vi "Frame Get i.vi"(8 "error in (no error)":errorcluster, 11 "IDE simple in":refnum<class "LF2R IDE.lvclass">) -> (0 "error out":errorcluster, 1 "<i> Data":T1, 2 "Iindex":u32, 3 "IDE simple out":refnum<class "LF2R IDE.lvclass">)   [LabVIEW 2018, in "LF2R IDE.lvlib" / "LF2R IDE.lvclass"]
uses:
  LF2R IDE.lvclass
  Frame Analizer/frame i data.ctl
  LF2R IDE.lvclass/LF2R IDE.ctl
  Frame Analizer/Data Parser.lvclass
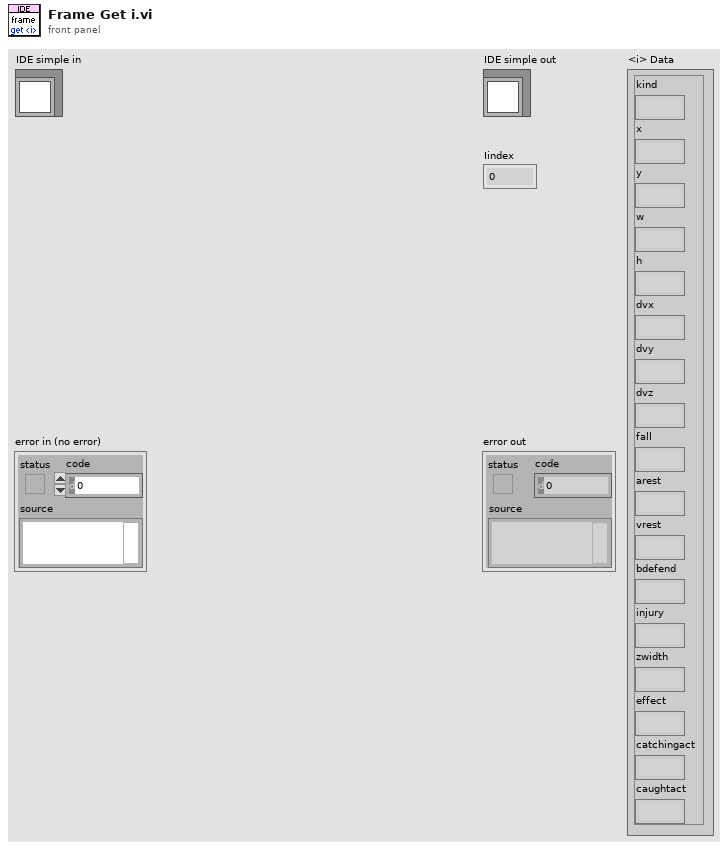
[diagram p1: front panel]
types:
  T1 = typedef "Data Parser.lvclass/frame i data.ctl" = cluster{"kind":string, "x":string, "y":string, "w":string, "h":string, "dvx":string, "dvy":string, "dvz":string, "fall":string, "arest":string, "vrest":string, "bdefend":string, "injury":string, "zwidth":string, "effect":string, "catchingact":string, "caughtact":string}
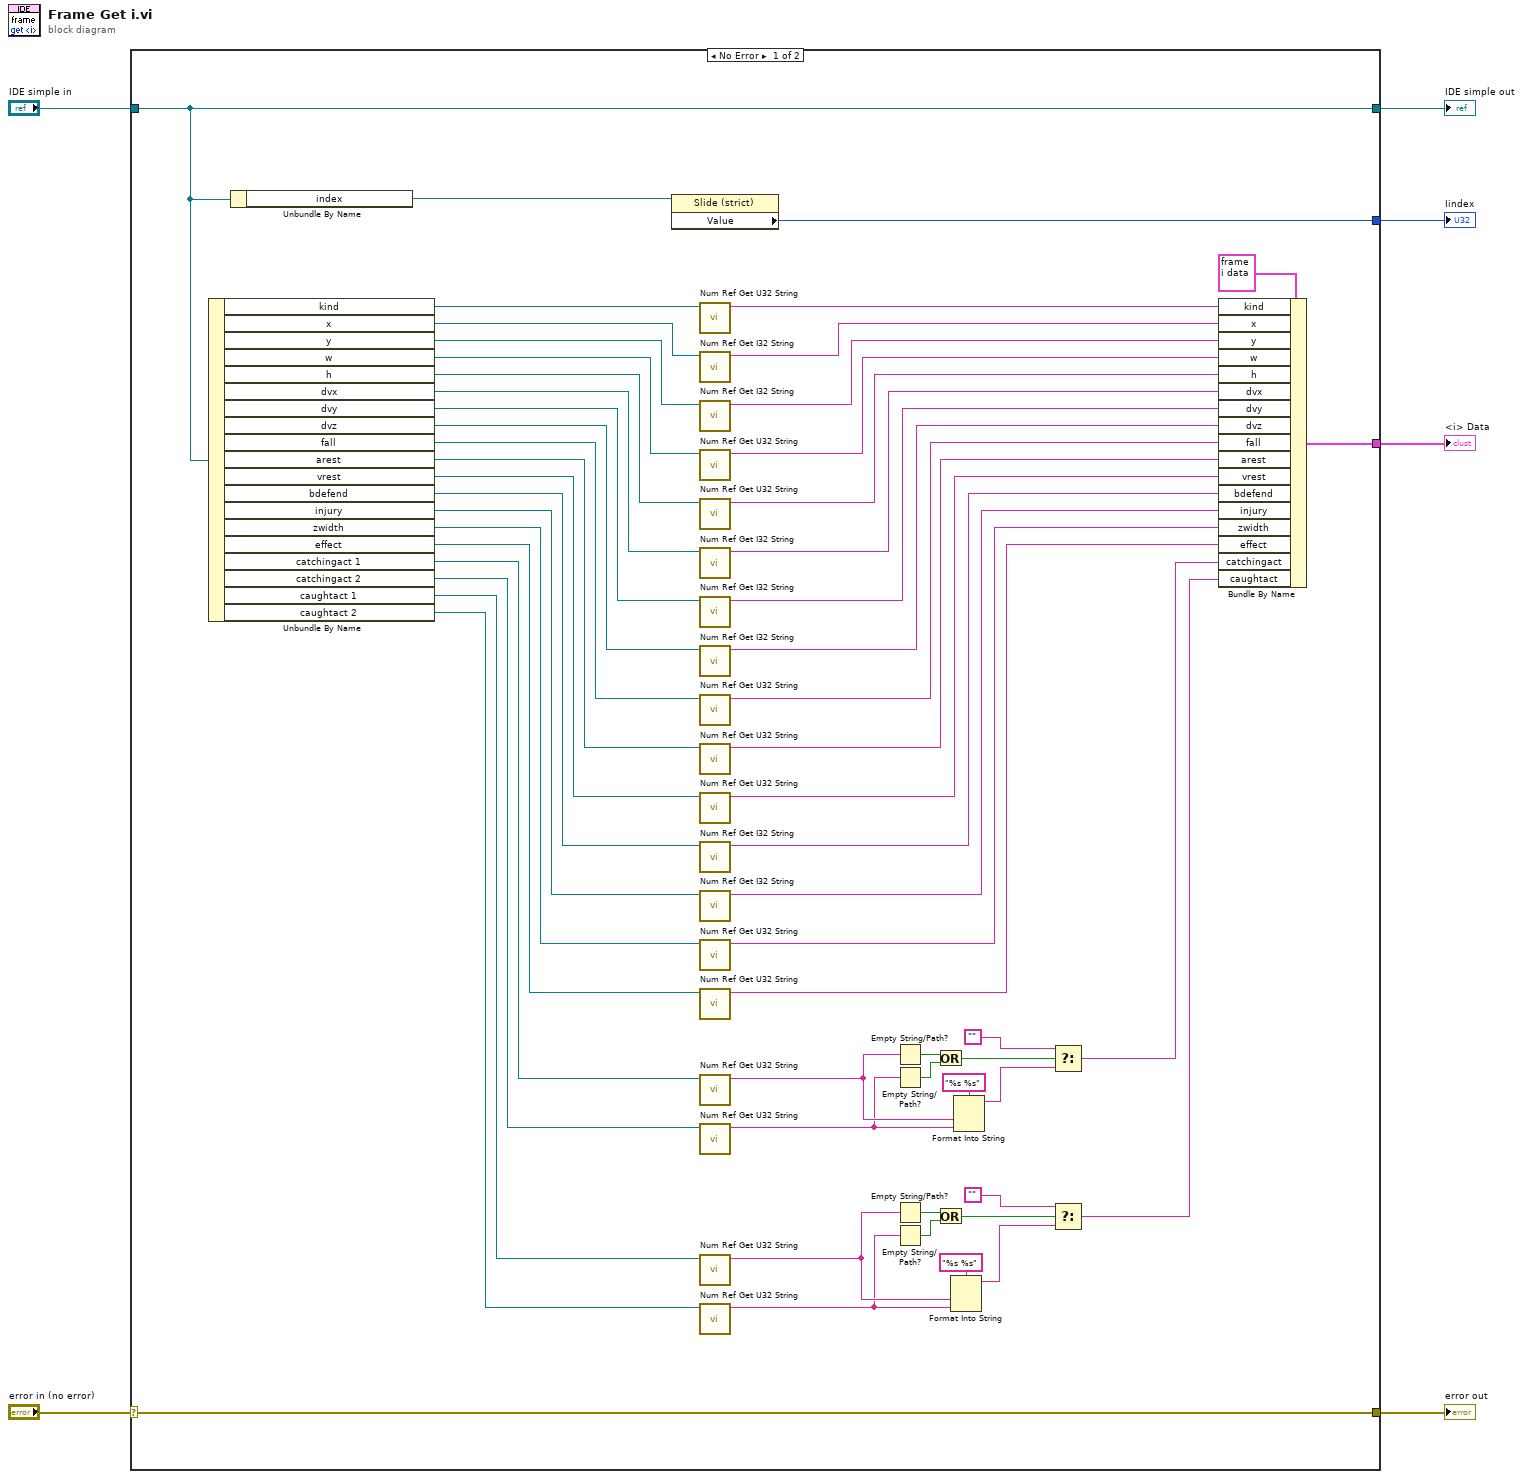
[diagram p0: block diagram]
diagram:
  n1 = case shown="No Error" "error in (no error)" {
    selector: "error in (no error)" -> [w26 w66]
    tunnel: [w26 w66] -> w5
    tunnel: [w25 w65] -> w3
    tunnel: "IDE simple in" -> [w25 w65]
    tunnel: [w64 _] -> w2
    tunnel: [w23 _] -> w1
    frame No Error {
      n2 = Unbundle By Name(w25) -> ("kind"=w62:refnum<vi>, "x"=w60:refnum<vi>, "y"=w59:refnum<vi>, "w"=w58:refnum<vi>, "h"=w57:refnum<vi>, "dvx"=w52:refnum<vi>, "dvy"=w51:refnum<vi>, "dvz"=w50:refnum<vi>, "fall"=w49:refnum<vi>, "arest"=w48:refnum<vi>, "vrest"=w47:refnum<vi>, "bdefend"=w46:refnum<vi>, "injury"=w45:refnum<vi>, "zwidth"=w44:refnum<vi>, "effect"=w43:refnum<vi>, "catchingact 1"=w42:refnum<vi>, "catchingact 2"=w41:refnum<vi>, "caughtact 1"=w40:refnum<vi>, "caughtact 2"=w39:refnum<vi>)
      n3 = Unbundle By Name(w25) -> ("index"=w24:refnum<vi>)
      n4 = property class="Slide (strict)"(reference=w24) -> ("Value"=w23:u32)  [unwired: 1 in, 2 out]
      n5 = call "Num Ref Get U32 String.vi"("U32 Ref"=w62) -> ("Value string"=w61:string)  [unwired: 9 in, 1 out]
      n6 = call "Num Ref Get I32 String.vi"("I32 Ref"=w60) -> ("Value String"=w56:string)  [unwired: 9 in, 1 out]
      n7 = call "Num Ref Get I32 String.vi"("I32 Ref"=w59) -> ("Value String"=w55:string)  [unwired: 9 in, 1 out]
      n8 = call "Num Ref Get U32 String.vi"("U32 Ref"=w58) -> ("Value string"=w54:string)  [unwired: 9 in, 1 out]
      n9 = call "Num Ref Get U32 String.vi"("U32 Ref"=w57) -> ("Value string"=w53:string)  [unwired: 9 in, 1 out]
      n10 = call "Num Ref Get I32 String.vi"("I32 Ref"=w52) -> ("Value String"=w38:string)  [unwired: 9 in, 1 out]
      n11 = call "Num Ref Get I32 String.vi"("I32 Ref"=w51) -> ("Value String"=w37:string)  [unwired: 9 in, 1 out]
      n12 = call "Num Ref Get I32 String.vi"("I32 Ref"=w50) -> ("Value String"=w36:string)  [unwired: 9 in, 1 out]
      n13 = call "Num Ref Get U32 String.vi"("U32 Ref"=w49) -> ("Value string"=w35:string)  [unwired: 9 in, 1 out]
      n14 = call "Num Ref Get U32 String.vi"("U32 Ref"=w48) -> ("Value string"=w34:string)  [unwired: 9 in, 1 out]
      n15 = call "Num Ref Get U32 String.vi"("U32 Ref"=w47) -> ("Value string"=w33:string)  [unwired: 9 in, 1 out]
      n16 = call "Num Ref Get I32 String.vi"("I32 Ref"=w46) -> ("Value String"=w32:string)  [unwired: 9 in, 1 out]
      n17 = call "Num Ref Get I32 String.vi"("I32 Ref"=w45) -> ("Value String"=w31:string)  [unwired: 9 in, 1 out]
      n18 = call "Num Ref Get U32 String.vi"("U32 Ref"=w44) -> ("Value string"=w30:string)  [unwired: 9 in, 1 out]
      n19 = call "Num Ref Get U32 String.vi"("U32 Ref"=w43) -> ("Value string"=w29:string)  [unwired: 9 in, 1 out]
      n20 = call "Num Ref Get U32 String.vi"("U32 Ref"=w42) -> ("Value string"=w22:string)  [unwired: 9 in, 1 out]
      n21 = call "Num Ref Get U32 String.vi"("U32 Ref"=w41) -> ("Value string"=w21:string)  [unwired: 9 in, 1 out]
      n22 = call "Num Ref Get U32 String.vi"("U32 Ref"=w40) -> ("Value string"=w10:string)  [unwired: 9 in, 1 out]
      n23 = call "Num Ref Get U32 String.vi"("U32 Ref"=w39) -> ("Value string"=w9:string)  [unwired: 9 in, 1 out]
      n24 = Empty String/Path?(string/path=w22) -> (empty?=w20:bool)
      n25 = Empty String/Path?(string/path=w21) -> (empty?=w19:bool)
      n26 = Empty String/Path?(string/path=w10) -> (empty?=w11:bool)
      n27 = Empty String/Path?(string/path=w9) -> (empty?=w12:bool)
      n28 = Or(x=w20, y=w19) -> (x .or. y?=w18:bool)
      n29 = Or(x=w11, y=w12) -> (x .or. y?=w13:bool)
      n30 = Format Into String(format string="%s %s", w10, w9) -> (resulting string=w8:string)  [unwired: 2 in, 1 out]
      n31 = Format Into String(format string="%s %s", w22, w21) -> (resulting string=w16:string)  [unwired: 2 in, 1 out]
      n32 = Select(t="", s=w18, f=w16) -> (s? t:f=w15:string)
      n33 = Select(t="", s=w13, f=w8) -> (s? t:f=w7:string)
      n34 = Bundle By Name(cluster=T1 {"kind"="", "x"="", "y"="", "w"="", "h"="", "dvx"="", "dvy"="", "dvz"="", "fall"="", "arest"="", "vrest"="", "bdefend"="", "injury"="", "zwidth"="", "effect"="", "catchingact"="", "caughtact"=""} ("<i> data 2"), "kind"=w61, "x"=w56, "y"=w55, "w"=w54, "h"=w53, "dvx"=w38, "dvy"=w37, "dvz"=w36, "fall"=w35, "arest"=w34, "vrest"=w33, "bdefend"=w32, "injury"=w31, "zwidth"=w30, "effect"=w29, "catchingact"=w15, "caughtact"=w7) -> (w64:T1)
    }
    frame Error {
    }
  }
  "error out" <- w5
  "IDE simple out" <- w3
  "<i> Data" <- w2
  "Iindex" <- w1
